vi "SunplusDaily.vi"() -> ()   [LabVIEW 2012]
uses:
  <vilib>/Utility/NIReport.llb/NI_report.lvclass
  <vilib>/addons/database/Auxilliary.llb/DB Tools Cursor Type.ctl
  <vilib>/addons/database/Connection.llb/DB Tools Open Connec (Path).vi
  <vilib>/addons/database/Connection.llb/Conn Execute.vi
  <vilib>/addons/database/Recordset.llb/Rec Fetch Recordset Data (R).vi
  <vilib>/addons/database/Recordset.llb/Rec Destroy - Connection.vi
  <vilib>/addons/database/_DB Variant To Data/Database Variant To Data.xnode
  <vilib>/addons/database/NI_Database_API.lvlib
  <vilib>/Utility/NIReport.llb/Excel/NI_Excel.lvclass
panel:
  out "error out 2":errorcluster
  out "report out":refnum<class "NI_report.lvclass">
  in  "start (0, 0)":cluster{"start row":i32, "start column":i32}
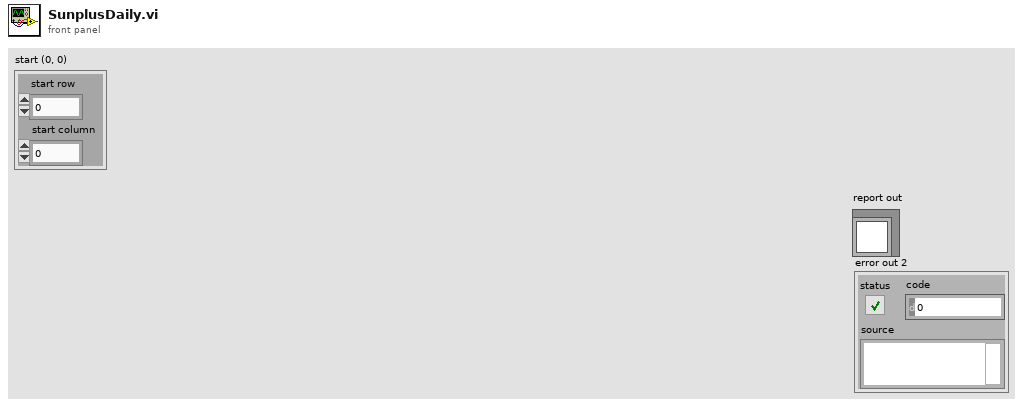
[diagram p1: front panel]
types:
  T1 = enum16{"Standard Report", "HTML", "Word", "Excel"}
  T2 = typedef "NI_Database_API.lvlib/DB Tools Cursor Type.ctl" = enum16{"forward-only", "keyset", "dynamic", "static"}
  T3 = typedef "NI_Database_API.lvlib/Conn ObjectReference.ctl" = refnum<k1>
  T4 = typedef "NI_Database_API.lvlib/Rec ObjectReference.ctl" = refnum<k1>
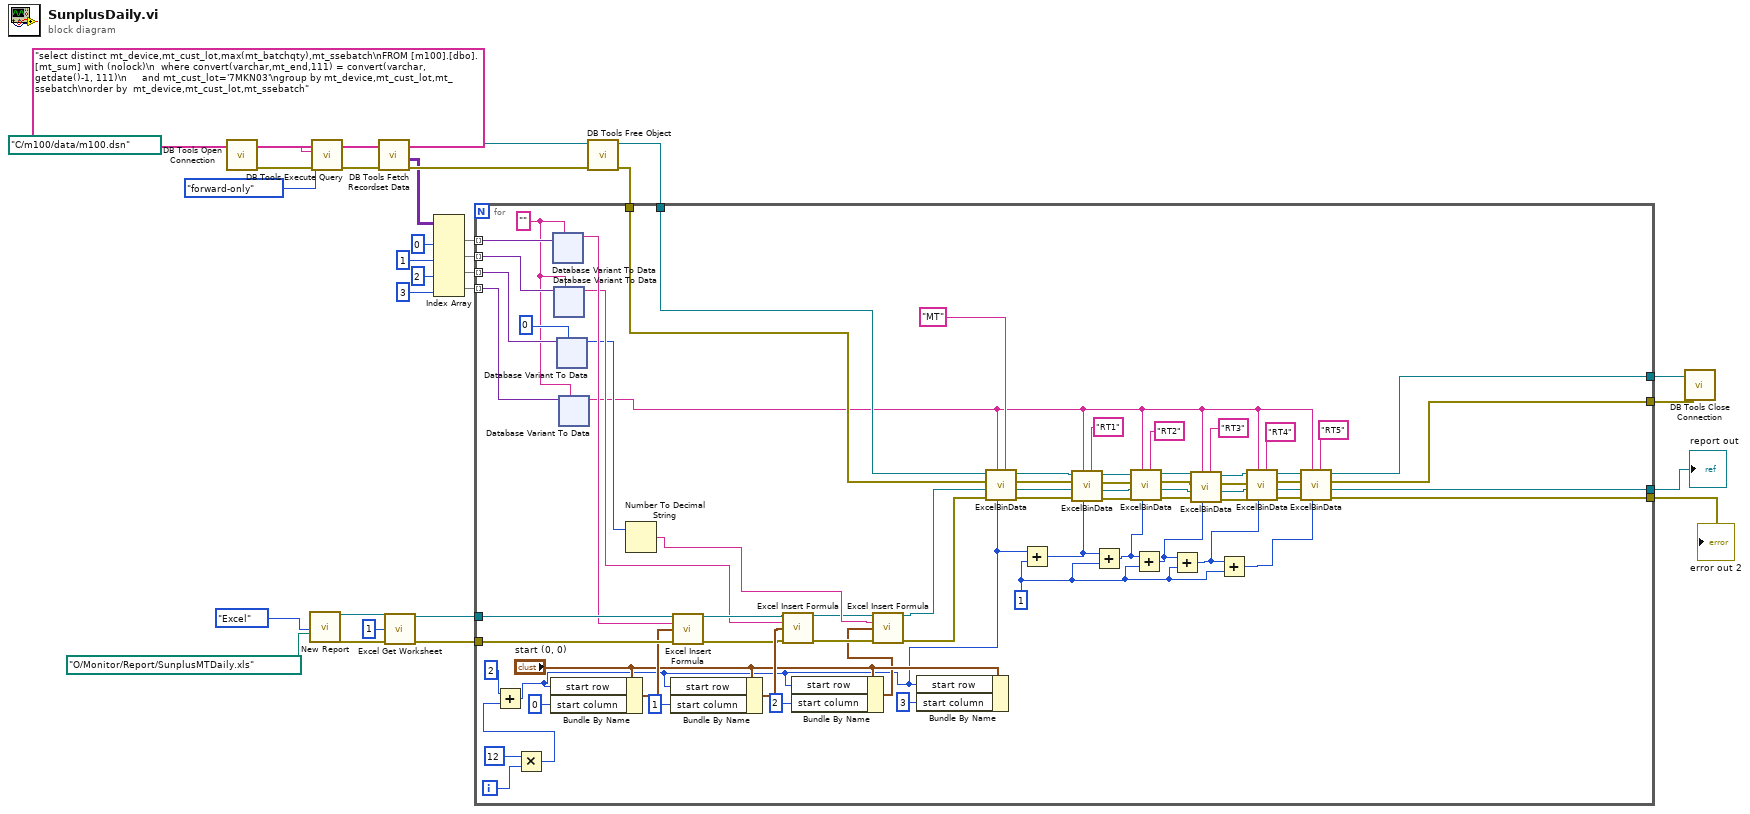
[diagram p0: block diagram]
diagram:
  n1 = call-poly <vilib>:"DB Tools Open Connection.vi"("connection information"=path "C:/m100/data/m100.dsn") -> ("error out"=w26:errorcluster, "connection reference"=w27:T3)  [unwired: 7 in]
  n2 = call <vilib>:"New Report.vi"("report type"=T1."Excel" ("Report Type"), "template (empty)"=path "O:/Monitor/Report/SunplusMTDaily.xls") -> ("report out"=w10:refnum<class "NI_report.lvclass">, "error out"=w9:errorcluster)  [unwired: 12 in]
  n3 = call-poly <vilib>:"DB Tools Execute Query.vi"("error in (no error)"=w26, "cursor type"=DB_Tools_Cursor_Type."forward-only", "SQL query"="select distinct mt_device,mt_cust_lot,max(mt_batchqty),mt_ssebatch\nFROM [m100].[dbo].[mt_sum] with (nolock)\n  where convert(varchar,mt_end,111) = convert(varchar, getdate()-1, 111)\n     and mt_cust_lot='7MKN03'\ngroup by mt_device,mt_cust_lot,mt_ssebatch\norder by  mt_device,mt_cust_lot,mt_ssebatch", "connection reference"=w27) -> ("error out"=w28:errorcluster, "recordset reference"=w29:T4)  [unwired: 4 in]
  n4 = call-poly <vilib>:"DB Tools Fetch Recordset Data.vi"("error in (no error)"=w28, "recordset reference"=w29) -> ("error out"=w30:errorcluster, "recordset data"=w22:variant[][], "recordset reference out"=w31:T4)  [unwired: 3 in]
  n5 = call <vilib>:"Excel Get Worksheet.vi"("report in"=w10, "worksheet index (0)"=1, "error in (no error)"=w9) -> ("report out"=w6:refnum<class "NI_report.lvclass">, "error out"=w5:errorcluster)  [unwired: 11 in]
  n6 = Index Array(array=w22, index (col) #1=0 ("disabled index (col)"), index (col) #2=1 ("index (col)"), index (col) #3=2 ("index (col)"), index (col) #4=3 ("index (col)")) -> (element #1=w18:variant[], element #2=w17:variant[], element #3=w16:variant[], element #4=w12:variant[])  [unwired: 4 in]
  n7 = call-poly <vilib>:"DB Tools Free Object.vi"("error in (no error)"=w30, "recordset reference"=w31) -> ("error out"=w15:errorcluster, "connection reference"=w14:T3)  [unwired: 8 in]
  n8 = for {
    tunnel: w18 -> [w101] mode=indexing
    tunnel: w17 -> [w100] mode=indexing
    tunnel: w16 -> [w99] mode=indexing
    tunnel: w15 -> [w76]
    tunnel: w14 -> [w77]
    tunnel: w12 -> [w97] mode=indexing
    tunnel: w6 -> [w95]
    tunnel: w5 -> [w94]
    tunnel: [w44] -> w2
    tunnel: [w43] -> w1
    tunnel: [w46] -> w4
    tunnel: [w45] -> w3
    i -> [w72]
    w39 = 1 ("y")
    w96 = ""
    n9 = Multiply(x=12, y=w72) -> (x*y=w70:i32)
    n10 = Add(x=2, y=w70) -> (x+y=w68:i32)
    n11 = Bundle By Name(cluster="start (0, 0)", "start row"=w68, "start column"=0) -> (w93:cluster{"start row":i32, "start column":i32})
    n12 = xnode "Database Variant To Data"("database variant"=w101, "type"=w96) -> ("data"=w90:string)  [unwired: 1 in, 1 out]
    n13 = xnode "Database Variant To Data"("database variant"=w100, "type"=w96) -> ("data"=w85:string)  [unwired: 1 in, 1 out]
    n14 = xnode "Database Variant To Data"("database variant"=w99, "type"=0) -> ("data"=w83:i32)  [unwired: 1 in, 1 out]
    n15 = xnode "Database Variant To Data"("database variant"=w97, "type"=w96) -> ("data"=w42:string)  [unwired: 1 in, 1 out]
    n16 = Number To Decimal String(number=w83) -> (decimal integer string=w82:string)  [unwired: 1 in]
    n17 = Bundle By Name(cluster="start (0, 0)", "start row"=w68, "start column"=1) -> (w88:cluster{"start row":i32, "start column":i32})
    n18 = call <vilib>:"Excel Insert Formula.vi"("report in"=w95, "formula"=w90, "start (0, 0)"=w93, "error in (no error)"=w94) -> ("report out"=w87:refnum<class "NI_report.lvclass">, "error out"=w86:errorcluster)  [unwired: 10 in]
    n19 = call <vilib>:"Excel Insert Formula.vi"("report in"=w87, "formula"=w85, "start (0, 0)"=w88, "error in (no error)"=w86) -> ("report out"=w81:refnum<class "NI_report.lvclass">, "error out"=w80:errorcluster)  [unwired: 10 in]
    n20 = Bundle By Name(cluster="start (0, 0)", "start row"=w68, "start column"=2) -> (w73:cluster{"start row":i32, "start column":i32})
    n21 = call <vilib>:"Excel Insert Formula.vi"("report in"=w81, "formula"=w82, "start (0, 0)"=w73, "error in (no error)"=w80) -> ("report out"=w75:refnum<class "NI_report.lvclass">, "error out"=w74:errorcluster)  [unwired: 10 in]
    n22 = Bundle By Name(cluster="start (0, 0)", "start row"=w68, "start column"=3) -> ()  [unwired: 1 out]
    n23 = call "ExcelBinData.vi"("step"="MT", "start row"=w68, "jobno"=w42, "error in (no error) 2"=w74, "report in"=w75, "error in (no error)"=w76, "connection reference 2"=w77) -> ("error out 2"=w64:errorcluster, "report out"=w65:refnum<class "NI_report.lvclass">, "error out"=w66:errorcluster, "connection reference"=w67:T3)  [unwired: 1 in]
    n24 = Add(x=w68, y=w39) -> (x+y=w41:i32)
    n25 = call "ExcelBinData.vi"("step"="RT1", "start row"=w41, "jobno"=w42, "error in (no error) 2"=w64, "report in"=w65, "error in (no error)"=w66, "connection reference 2"=w67) -> ("error out 2"=w59:errorcluster, "report out"=w60:refnum<class "NI_report.lvclass">, "error out"=w61:errorcluster, "connection reference"=w62:T3)  [unwired: 1 in]
    n26 = Add(x=w41, y=w39) -> (x+y=w40:i32)
    n27 = call "ExcelBinData.vi"("step"="RT2", "start row"=w40, "jobno"=w42, "error in (no error) 2"=w59, "report in"=w60, "error in (no error)"=w61, "connection reference 2"=w62) -> ("error out 2"=w55:errorcluster, "report out"=w56:refnum<class "NI_report.lvclass">, "error out"=w57:errorcluster, "connection reference"=w58:T3)  [unwired: 1 in]
    n28 = Add(x=w40, y=w39) -> (x+y=w34:i32)
    n29 = Add(x=w34, y=w39) -> (x+y=w33:i32)
    n30 = call "ExcelBinData.vi"("step"="RT3", "start row"=w34, "jobno"=w42, "error in (no error) 2"=w55, "report in"=w56, "error in (no error)"=w57, "connection reference 2"=w58) -> ("error out 2"=w51:errorcluster, "report out"=w52:refnum<class "NI_report.lvclass">, "error out"=w53:errorcluster, "connection reference"=w54:T3)  [unwired: 1 in]
    n31 = Add(x=w33, y=w39) -> (x+y=w32:i32)
    n32 = call "ExcelBinData.vi"("step"="RT4", "start row"=w33, "jobno"=w42, "error in (no error) 2"=w51, "report in"=w52, "error in (no error)"=w53, "connection reference 2"=w54) -> ("error out 2"=w47:errorcluster, "report out"=w48:refnum<class "NI_report.lvclass">, "error out"=w49:errorcluster, "connection reference"=w50:T3)  [unwired: 1 in]
    n33 = call "ExcelBinData.vi"("step"="RT5", "start row"=w32, "jobno"=w42, "error in (no error) 2"=w47, "report in"=w48, "error in (no error)"=w49, "connection reference 2"=w50) -> ("error out 2"=w43:errorcluster, "report out"=w44:refnum<class "NI_report.lvclass">, "error out"=w45:errorcluster, "connection reference"=w46:T3)  [unwired: 1 in]
  }
  "report out" <- w2
  "error out 2" <- w1
  n34 = call <vilib>:"DB Tools Close Connection.vi"("error in (no error)"=w3, "connection reference"=w4) -> ()  [unwired: 5 in, 1 out]
